vi "poly_sub(s)_filter.vi"(8 "error in (no error)":errorcluster, 9 "f":i32=50 caption="base frequency (50Hz)", 10 "N":i32=3 caption="N of harmonics to remove (3)", 11 "xwave in":T1={"attributes"=variant, "X"={"start"=0.0, "delta"=0.0, "units"="index", "dim"="au"}, "Y"={"data"=[], "units"="au"}}) -> (0 "error out":errorcluster, 3 "xwave out":T1={"attributes"=variant, "X"={"start"=0.0, "delta"=0.0, "units"="index", "dim"="au"}, "Y"={"data"=[], "units"="au"}})   [LabVIEW 2015]
uses:
  xwave/xwav.ctl
  <vilib>/measure/matone.llb/Extract Single Tone Information 1 Chan.vi
  <vilib>/measure/NI_MAPro.lvlib
  <vilib>/Analysis/NI_AALBase.lvlib
panel:
  out "Automatic line filter level detection":cluster{dbl[], dbl[]}[](graph)
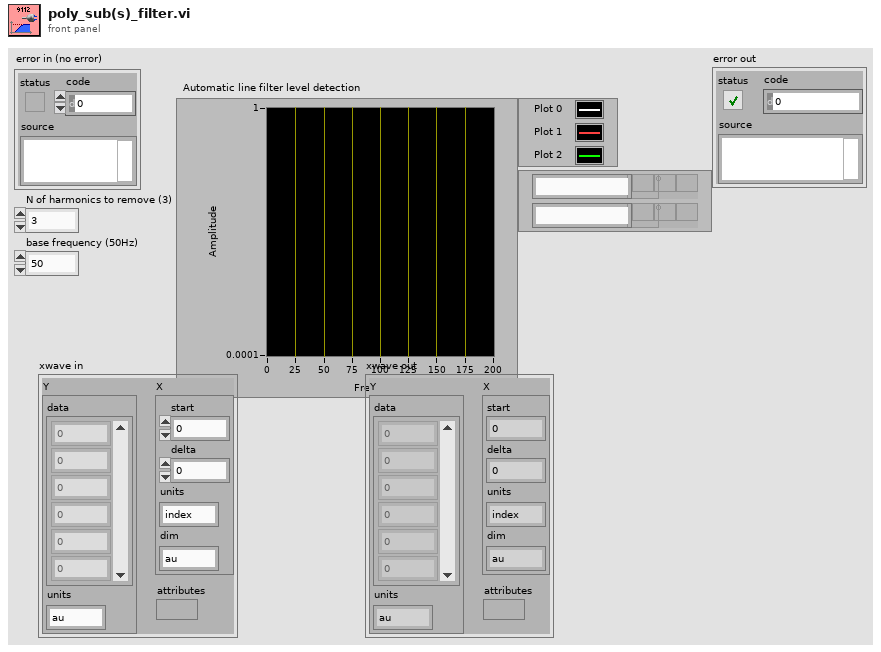
[diagram p1: front panel]
types:
  T1 = typedef "xwav.ctl" = cluster{"attributes":variant, "X":cluster{"start":dbl, "delta":dbl, "units":string, "dim":string}, "Y":cluster{"data":dbl[], "units":string}}
  T2 = cluster{"approx freq. (optional)":dbl, "search (+/- % of Fsampl.)":dbl}
  T3 = enum32{"none", "input signal", "detected signal", "residual signal"}
  T4 = cluster{"exported time signal":waveform(dbl), "exported spectrum (dB)":cluster{"f0":dbl, "df":dbl, "dB Spectrum (Hann)":dbl[]}}
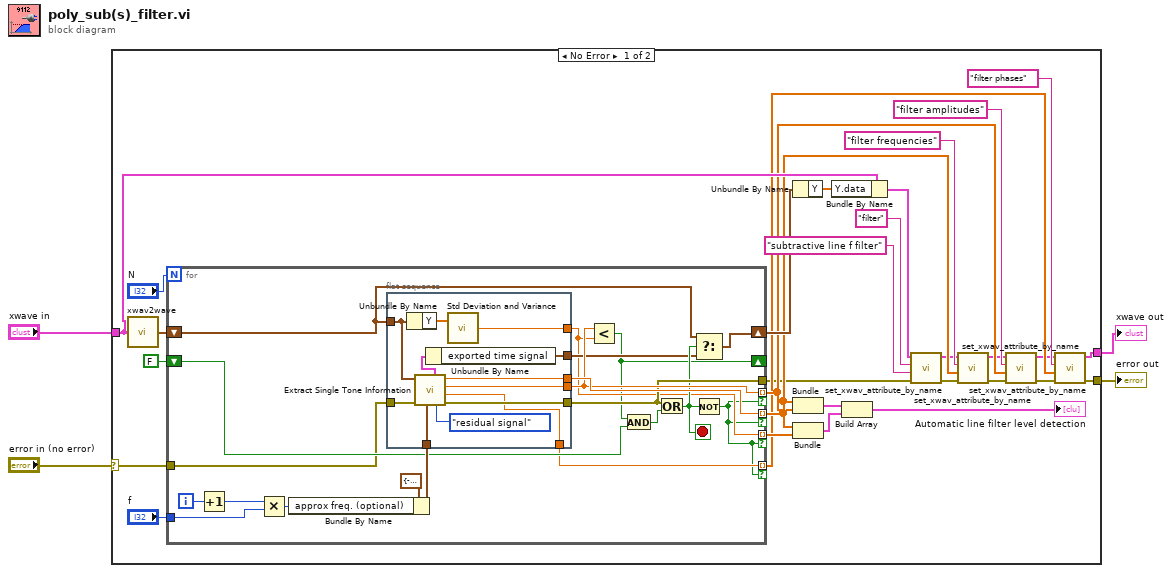
[diagram p0: block diagram]
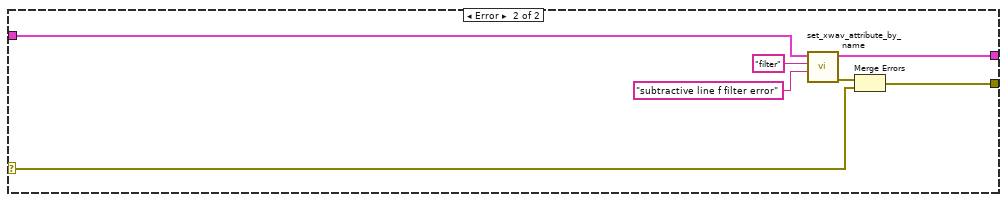
[diagram p2: hidden frame]
diagram:
  n1 = case shown="No Error" "error in (no error)" {
    selector: "error in (no error)" -> [w29 w68]
    tunnel: [w5 w67] -> w4
    tunnel: [w10 w70] -> w1
    tunnel: "xwave in" -> [w23 w71]
    frame No Error {
      n2 = call "xwav2wave.vi"("xwave"=w23) -> ("waveform"=w26:waveform(dbl))  [unwired: 4 in]
      n3 = for {
        N: "N" -> [_]
        shift-right: [w46] -> w25
        shift-left: w26 -> [w43]
        tunnel: [w54] -> w18 mode=indexing if=w35
        tunnel: [w47] -> w9
        tunnel: [w48] -> w16 mode=indexing if=w35
        tunnel: [w42] -> w33 mode=indexing if=w35
        shift-right: [w40] -> _
        shift-left: FALSE -> [w41]
        tunnel: w29 -> [w38]
        tunnel: "f" -> [w37]
        tunnel: [w36] -> w14 mode=indexing if=w35
        i -> [w51]
        stop <- w45 stop-if-true
        n4 = Increment(x=w51) -> (x+1=w50:i32)
        n5 = Multiply(x=w50, y=w37) -> (x*y=w49:i32)
        n6 = Bundle By Name(cluster=T2 {"approx freq. (optional)"=-1.0, "search (+/- % of Fsampl.)"=5.0} ("advanced search"), "approx freq. (optional)"=w49) -> (w52:T2)
        n7 = flat-sequence {
          tunnel: [w65] -> w54
          tunnel: w52 -> [w64]
          tunnel: [w63] -> w48
          tunnel: [w62] -> w47
          tunnel: [w60] -> w44
          tunnel: w43 -> [w58]
          tunnel: [w57] -> w42
          tunnel: w38 -> [w56]
          tunnel: [w55] -> w36
          frame #0 {
            n8 = Unbundle By Name(w58) -> ("Y"=w61:dbl[])
            n9 = call-poly <vilib>:"Extract Single Tone Information.vi"("advanced search"=w64, "error in (no error)"=w56, "export mode"=T3."residual signal", "time signal in"=w58) -> ("error out"=w62:errorcluster, "detected phase (deg)"=w55:dbl, "detected amplitude"=w63:dbl, "detected frequency"=w65:dbl, "exported signals"=w59:T4)  [unwired: 2 in, 1 out]
            n10 = Unbundle By Name(w59) -> ("exported time signal"=w60:waveform(dbl))
            n11 = call <vilib>:"Std Deviation and Variance.vi"("X"=w61) -> ("standard deviation"=w57:dbl)  [unwired: 1 in, 2 out]
          }
        }
        n12 = Less?(x=w48, y=w42) -> (x < y?=w40:bool)
        n13 = And(x=w40, y=w41) -> (x .and. y?=w39:bool)
        n14 = Or(x=w47, y=w39) -> (x .or. y?=w45:bool)
        n15 = Select(t=w43, s=w45, f=w44) -> (s? t:f=w46:waveform(dbl))
        n16 = Not(x=w45) -> (.not. x?=w35:bool)
      }
      n17 = Unbundle By Name(w25) -> ("Y"=w24:dbl[])
      n18 = Bundle(w18, w16) -> (w32:cluster{dbl[], dbl[]})  [unwired: 1 in]
      n19 = Bundle(w18, w33) -> (w31:cluster{dbl[], dbl[]})  [unwired: 1 in]
      n20 = Bundle By Name(cluster=w23, "Y.data"=w24) -> (w20:T1)
      n21 = Build Array(w32, w31) -> (→"Automatic line filter level detection":cluster{dbl[], dbl[]}[])
      n22 = call "set_xwav_attribute_by_name.vi"("Error in"=w9, "value"="subtractive line f filter" ("name"), "name"="filter", "xwave in"=w20) -> ("Error out"=w8:errorcluster, "xwave out"=w13:T1)  [unwired: 5 in, 1 out]
      n23 = call "set_xwav_attribute_by_name.vi"("Error in"=w8, "value"=w18, "name"="filter frequencies", "xwave in"=w13) -> ("Error out"=w7:errorcluster, "xwave out"=w12:T1)  [unwired: 5 in, 1 out]
      n24 = call "set_xwav_attribute_by_name.vi"("Error in"=w7, "value"=w16, "name"="filter amplitudes", "xwave in"=w12) -> ("Error out"=w6:errorcluster, "xwave out"=w11:T1)  [unwired: 5 in, 1 out]
      n25 = call "set_xwav_attribute_by_name.vi"("Error in"=w6, "value"=w14, "name"="filter phases", "xwave in"=w11) -> ("Error out"=w5:errorcluster, "xwave out"=w10:T1)  [unwired: 5 in, 1 out]
    }
    frame Error {
      n26 = call "set_xwav_attribute_by_name.vi"("value"="subtractive line f filter error" ("name"), "name"="filter", "xwave in"=w71) -> ("Error out"=w69:errorcluster, "xwave out"=w70:T1)  [unwired: 6 in, 1 out]
      n27 = Merge Errors(w69, w68) -> (w67:errorcluster)
    }
  }
  "error out" <- w4
  "xwave out" <- w1
